vi "MSGraph Component Check.vi"(1 "error 2":errorcluster, 2 "error 1":errorcluster, 3 "MS Graph":refnum<k7>) -> (0 "error out":errorcluster)   [LabVIEW 2020, in "NI_ReportGenerationToolkit.lvlib"]
uses:
  <vilib>/addons/_office/NI_ReportGenerationToolkit.lvlib
  <vilib>/Utility/NIReport.llb/NI_ReportGenerationCore.lvlib
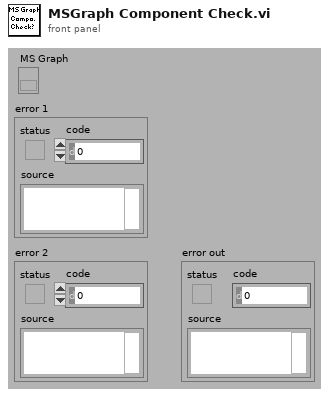
[diagram p1: front panel]
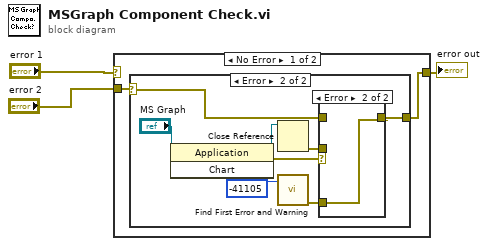
[diagram p0: block diagram]
diagram:
  n1 = case shown="No Error" "error 1" {
    selector: "error 1" -> [_ w17]
    tunnel: [w4 w17] -> w2
    tunnel: "error 2" -> [w5 _]
    frame No Error {
      n2 = case shown="Error" w5 {
        selector: w5 -> [w6 w8]
        tunnel: [w6 w9] -> w4
        frame No Error {
        }
        frame Error {
          n3 = invoke class="Application" method="Chart"(reference="MS Graph") -> (reference out=w13:refnum<k7>, error out=w11:errorcluster)  [unwired: 2 in, 1 out]
          n4 = Close Reference(reference=w13) -> (error out=w7:errorcluster)  [unwired: 1 in]
          n5 = call <vilib>:"Find First Error and Warning.vi"("error code"=-41105 ("code")) -> ("error out"=w10:errorcluster)  [unwired: 1 in, 5 out]
          n6 = case shown="Error" w11 {
            tunnel: w10 -> [_ w16]
            tunnel: [w15 w16] -> w9
            tunnel: w8 -> [w15 _]
            tunnel: w7 -> [_ _]
            frame No Error {
            }
            frame Error {
            }
          }
        }
      }
    }
    frame Error {
    }
  }
  "error out" <- w2
